vi "labview截图稳定快速版.vi"() -> ()   [LabVIEW 2018]
uses:
  PrtScToByte.dll
panel:
  out "x-y":u32
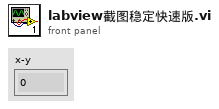
[diagram p1: front panel]
types:
  T1 = typedef "IMAQ Image.ctl" = refnum<image>
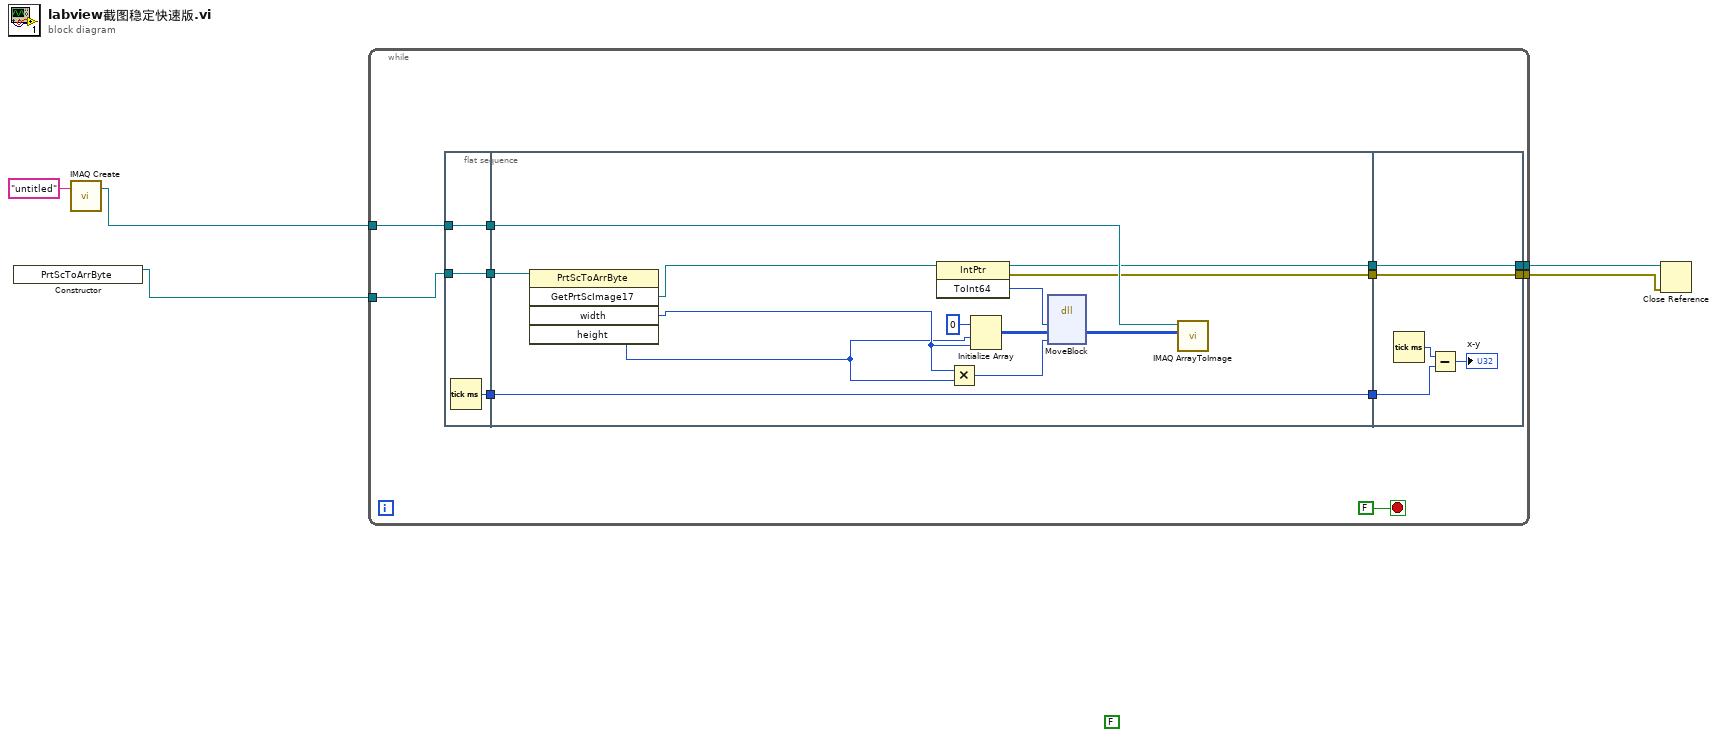
[diagram p0: block diagram]
diagram:
  (unwired) FALSE
  n1 = constructor class="PrtScToArrByte"() -> (reference out=w2:refnum<k24>)  [unwired: 3 in, 2 out]
  n2 = call "IMAQ Create"("Image Name"="untitled") -> ("New Image"=w5:T1)  [unwired: 4 in, 1 out]
  n3 = while {
    tunnel: w5 -> [w16]
    tunnel: [w15] -> w3
    tunnel: w2 -> [w13]
    tunnel: [w12] -> w1
    stop <- FALSE stop-if-true
    n4 = flat-sequence {
      tunnel: w13 -> [w18]
      tunnel: w16 -> [w19]
      tunnel: [w19] -> w11
      tunnel: [w18] -> w10
      tunnel: [w17] -> w6
      tunnel: w11 -> [w32]
      tunnel: w10 -> [w30]
      tunnel: [w31] -> w9
      tunnel: [w21] -> w8
      tunnel: [w20] -> w7
      tunnel: w6 -> [w20]
      tunnel: [w36] -> w12
      tunnel: [w37] -> w15
      tunnel: w9 -> [w37]
      tunnel: w8 -> [w36]
      tunnel: w7 -> [w33]
      frame #0 {
        n5 = Tick Count (ms)() -> (millisecond timer value=w17:u32)
      }
      frame #1 {
        n6 = invoke on="调用节点" class="PrtScToArrByte" method="GetPrtScImage17"(reference=w30) -> ("GetPrtScImage17"=w27:refnum<k24>, "width"=w29:i32, "height"=w28:i32)  [unwired: 4 in, 2 out]
        n7 = invoke on="调用节点" class="IntPtr" method="ToInt64"(reference=w27) -> (reference out=w21:refnum<k24>, error out=w31:errorcluster, "ToInt64"=w23:i64)  [unwired: 2 in]
        n8 = Multiply(x=w29, y=w28) -> (x*y=w24:i32)
        n9 = Initialize Array(u8 0 ("element"), w28, w29) -> (w25:u8[][])
        n10 = dll-call lib="LabVIEW" fn="MoveBlock"("Source"=w23, "Dest"=w25, "Size"=w24) -> ("Dest"=w22:u8[][])  [unwired: 6 in, 2 out]
        n11 = call "IMAQ ArrayToImage"("Image Pixels (U8)"=w22, "Image"=w32) -> ()  [unwired: 8 in, 2 out]
      }
      frame #2 {
        n12 = Tick Count (ms)() -> (millisecond timer value=w34:u32)
        n13 = Subtract(x=w34, y=w33) -> (x-y=→"x-y":u32)
      }
    }
  }
  n14 = Close Reference(reference=w1, error in (no error)=w3) -> ()  [unwired: 1 out]
